vi "倒计时器.vi"() -> ()   [LabVIEW 2017]
panel:
  in  "定时时间选择":enum16{"20秒", "10秒", "6秒"}(ring)
  in  "开始倒计时":bool
  out "倒计时":string
  out "布尔":bool
  in  "停止":bool
  # "倒  计  时  器"
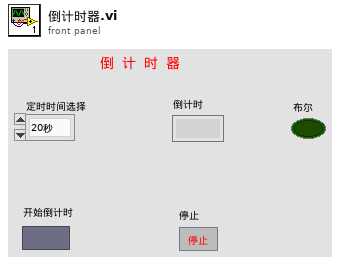
[diagram p1: front panel]
types:
  T1 = enum8{"Enabled", "Disabled", "Disabled and Grayed Out"}
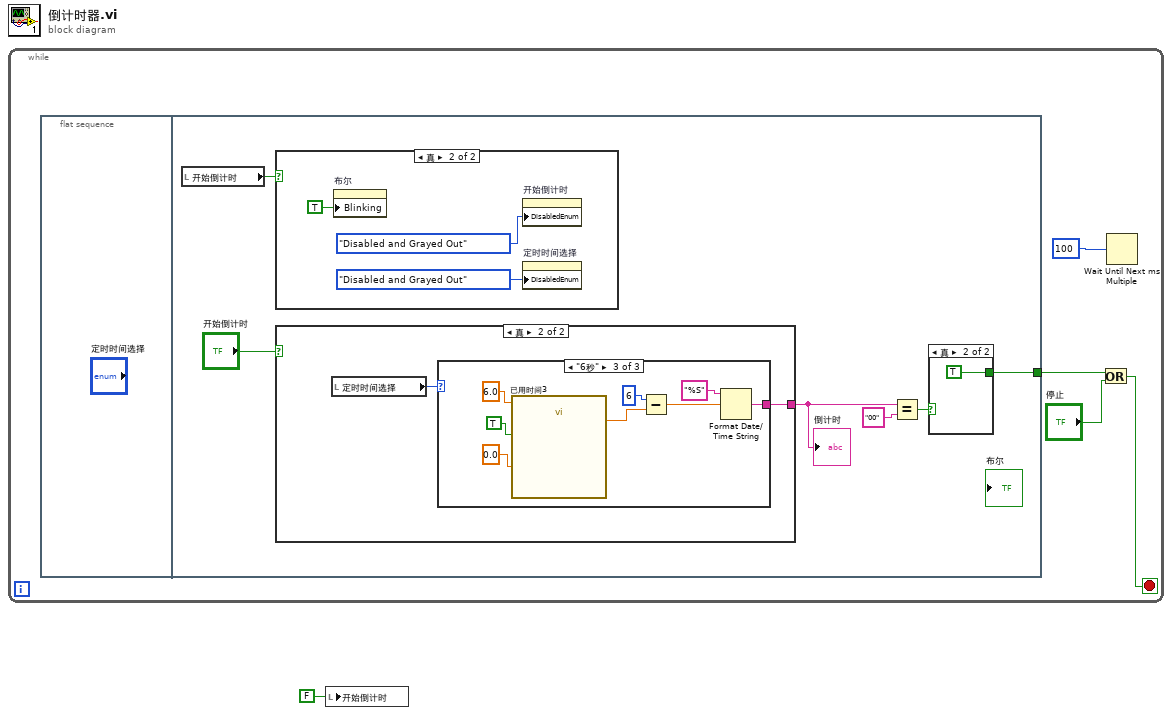
[diagram p0: block diagram]
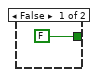
[diagram p2: hidden frame]
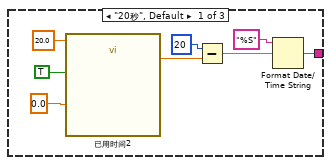
[diagram p4: hidden frame]
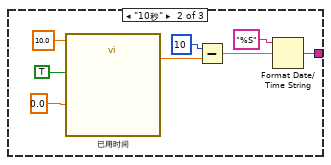
[diagram p5: hidden frame]
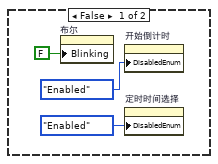
[diagram p6: hidden frame]
diagram:
  n1 = while {
    stop <- w2 stop-if-true
    n2 = flat-sequence {
      tunnel: [w9] -> w4
      frame #0 {
      }
      frame #1 {
        n3 = local read "开始倒计时"() -> (w10:bool)
        n4 = case shown="真" w10 {
          frame False {
            n5 = property on="布尔" class="Bool (严格)"("Blinking"=FALSE ("闪烁")) -> ()  [unwired: 2 in, 2 out]
            n6 = property on="开始倒计时" class="Bool (严格)"("DisabledEnum"=T1."Enabled" ("禁用")) -> ()  [unwired: 2 in, 2 out]
            n7 = property on="定时时间选择" class="Enum (严格)"("DisabledEnum"=T1."Enabled" ("禁用")) -> ()  [unwired: 2 in, 2 out]
          }
          frame True {
            n8 = property on="布尔" class="Bool (严格)"("Blinking"=TRUE ("闪烁")) -> ()  [unwired: 2 in, 2 out]
            n9 = property on="开始倒计时" class="Bool (严格)"("DisabledEnum"=T1."Disabled and Grayed Out" ("禁用")) -> ()  [unwired: 2 in, 2 out]
            n10 = property on="定时时间选择" class="Enum (严格)"("DisabledEnum"=T1."Disabled and Grayed Out" ("禁用")) -> ()  [unwired: 2 in, 2 out]
          }
        }
        n11 = case shown="真" "开始倒计时" {
          tunnel: [_ w15] -> w8
          frame False {
          }
          frame True {
            n12 = local read "定时时间选择"() -> (w14:enum16{"20秒", "10秒", "6秒"})
            n13 = case shown="\"6秒\"" w14 {
              tunnel: [w21 w29 w37] -> w15
              frame "20秒", Default {
                n14 = call "已用时间2"("Time Target (s)"=20.0, "Auto Reset"=TRUE, "Set Start Time (s)"=0.0) -> ("Elapsed Time (s)"=w18:dbl)  [unwired: 9 in, 7 out]
                n15 = Subtract(x=20, y=w18) -> (x-y=w17:dbl)
                n16 = Format Date/Time String(time format string (%c)="%S" ("时间格式字符串(%c)"), seconds (now)=w17) -> (date/time string=w21:string)  [unwired: 1 in]
              }
              frame "10秒" {
                n17 = call "已用时间"("Time Target (s)"=10.0, "Auto Reset"=TRUE, "Set Start Time (s)"=0.0) -> ("Elapsed Time (s)"=w26:dbl)  [unwired: 9 in, 7 out]
                n18 = Subtract(x=10, y=w26) -> (x-y=w25:dbl)
                n19 = Format Date/Time String(time format string (%c)="%S" ("时间格式字符串(%c)"), seconds (now)=w25) -> (date/time string=w29:string)  [unwired: 1 in]
              }
              frame "6秒" {
                n20 = call "已用时间3"("Time Target (s)"=6.0, "Auto Reset"=TRUE, "Set Start Time (s)"=0.0) -> ("Elapsed Time (s)"=w34:dbl)  [unwired: 9 in, 7 out]
                n21 = Subtract(x=6, y=w34) -> (x-y=w33:dbl)
                n22 = Format Date/Time String(time format string (%c)="%S" ("时间格式字符串(%c)"), seconds (now)=w33) -> (date/time string=w37:string)  [unwired: 1 in]
              }
            }
          }
        }
        "倒计时" <- w8
        n23 = Equal?(x=w8, y="00") -> (x = y?=w6:bool)
        n24 = case shown="真" w6 {
          tunnel: [FALSE TRUE] -> w9
          frame False {
          }
          frame True {
          }
        }
      }
    }
    n25 = Or(x=w4, y="停止") -> (x .or. y?=w2:bool)
    n26 = Wait Until Next ms Multiple(millisecond multiple=u32 100 ("毫秒倍数")) -> ()  [unwired: 1 out]
  }
  n27 = local write "开始倒计时"(FALSE ("开始倒计时")) -> ()
